vi "DrawMove.vi"(4 "Arena Pixel Dim":i32[](array[numeric])=[1000, 512], 6 "Show Vectors?":bool, 7 "Move":T1, 8 "picture in":picture) -> (3 "picture out":picture)   [LabVIEW 2015, in "MissionControl2017.lvlib"]
uses:
  MissionControl2017.lvlib
  Move.ctl
  Navigation2017.lvlib
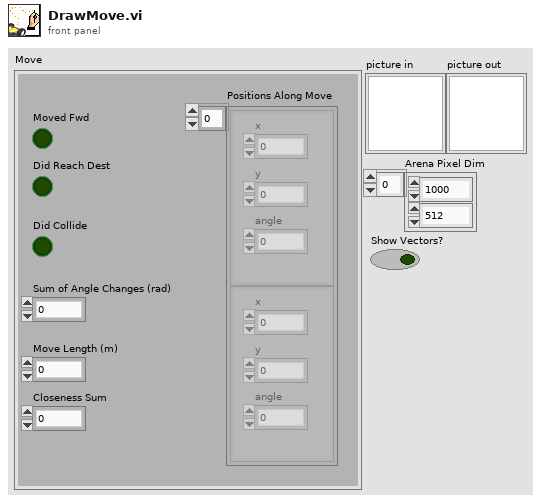
[diagram p1: front panel]
types:
  T1 = typedef "Navigation2017.lvlib/Move.ctl" = cluster{"Did Reach Dest":bool, "Did Collide":bool, "Sum of Angle Changes (rad)":dbl, "Move Length (m)":dbl, "Closeness Sum":dbl, "Positions Along Move":cluster{"x":dbl, "y":dbl, "angle":dbl}[], "Moved Fwd":bool}
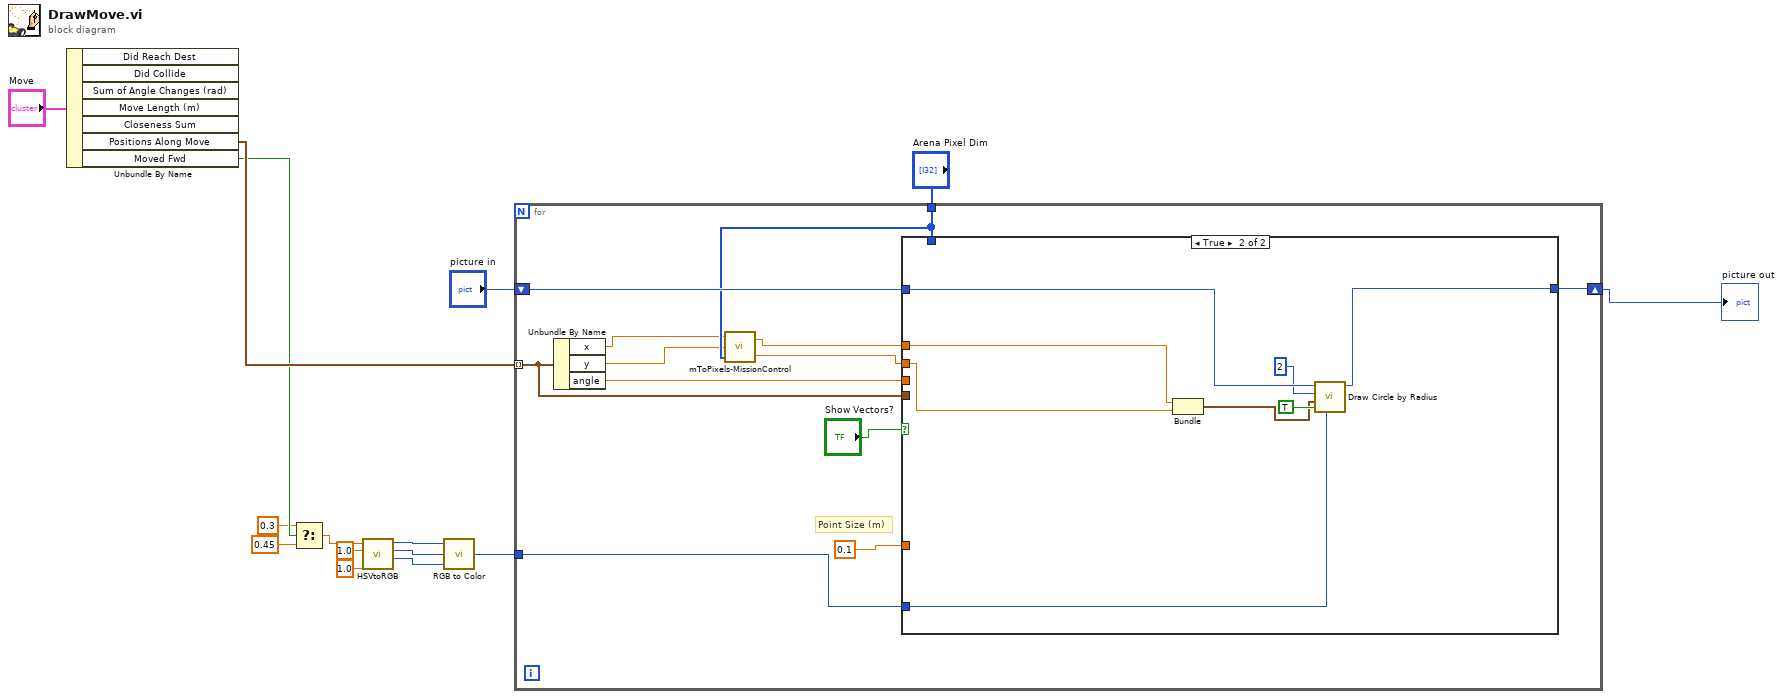
[diagram p0: block diagram]
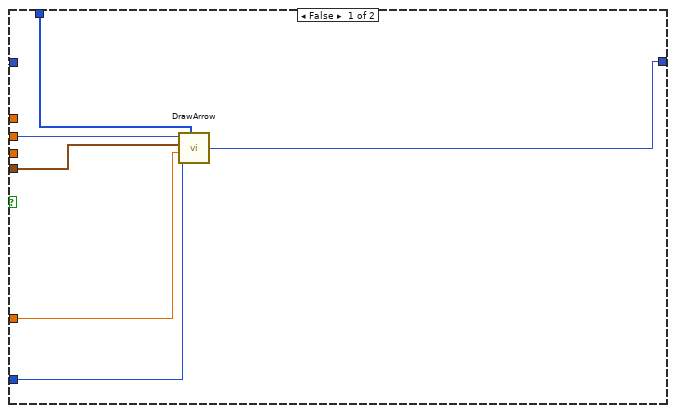
[diagram p2: hidden frame]
diagram:
  n1 = Unbundle By Name("Move") -> ("Positions Along Move"=w14:cluster{"x":dbl, "y":dbl, "angle":dbl}[], "Moved Fwd"=w3:bool)  [unwired: 5 out]
  n2 = Select(t=0.3, s=w3, f=0.45) -> (s? t:f=w6:dbl)
  n3 = call "HSVtoRGB.vi"("Value"=1.0, "Saturation"=1.0, "Hue [0-1)"=w6) -> ("Blue"=w10:u8, "Green"=w9:u8, "Red"=w8:u8)  [unwired: 6 in]
  n4 = call <vilib>:"RGB to Color.vi"("B"=w10, "G"=w9, "R"=w8) -> ("Color"=w7:u32)
  n5 = for {
    tunnel: w14 -> [w22] mode=indexing
    shift-right: [w26] -> w12
    shift-left: "picture in" -> [w27]
    tunnel: "Arena Pixel Dim" -> [w18]
    tunnel: w7 -> [w21]
    # "Point Size (m)"
    n6 = Unbundle By Name(w22) -> ("x"=w16:dbl, "y"=w17:dbl, "angle"=w24:dbl)
    n7 = call "mToPixels-MissionControl.vi"("Arena Pixel Dim"=w18, "y (m)"=w17, "x (m)"=w16) -> ("y (pixels)"=w19:dbl, "x (pixels)"=w20:dbl)
    n8 = case shown="True" "Show Vectors?" {
      tunnel: w27 -> [w33 w38]
      tunnel: [w32 w39] -> w26
      tunnel: w20 -> [_ w35]
      tunnel: w19 -> [_ w34]
      tunnel: w24 -> [_ _]
      tunnel: w18 -> [w31 _]
      tunnel: 0.1 ("y (m)") -> [w30 _]
      tunnel: w21 -> [w28 w40]
      tunnel: w22 -> [w29 _]
      frame False {
        n9 = call "DrawArrow.vi"("Arena Pixel Dim"=w31, "Color"=w28, "Length (m)"=w30, "Vector (m)"=w29, "picture"=w33) -> ("new picture"=w32:picture)  [unwired: 1 in]
      }
      frame True {
        n10 = Bundle("x (pixels)"=w35, "y (pixels)"=w34) -> (w36:cluster{"x (pixels)":dbl, "y (pixels)":dbl})  [unwired: 1 in]
        n11 = call <vilib>:"Draw Circle by Radius.vi"("color(black)"=w40, "fill?(F)"=TRUE, "pixel center"=w36, "radius"=i16 2, "picture"=w38) -> ("new picture"=w39:picture)  [unwired: 6 in]
      }
    }
  }
  "picture out" <- w12
